vi "FGV.vi"(7 "State":enum16{"Set", "Get"}(ring)) -> (3 "Data Output":dbl)   [LabVIEW 2019]
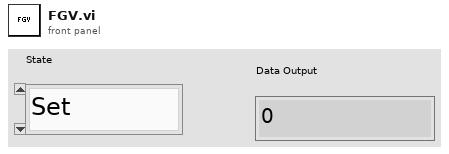
[diagram p1: front panel]
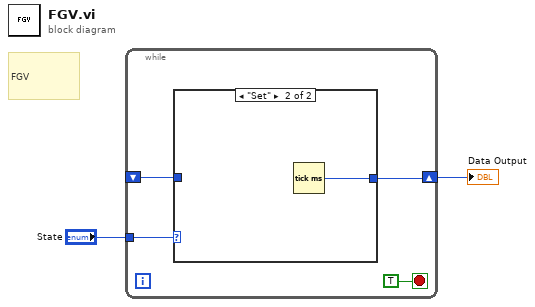
[diagram p0: block diagram]
diagram:
  # "FGV"
  n1 = while {
    shift-right: [w4] -> w1
    shift-left: _ -> [w3]
    tunnel: "State" -> [w5]
    stop <- TRUE stop-if-true
    n2 = case shown="\"Set\"" w5 {
      tunnel: [w7 w8] -> w4
      tunnel: w3 -> [w7 _]
      frame "Get" {
      }
      frame "Set" {
        n3 = Tick Count (ms)() -> (millisecond timer value=w8:u32)
      }
    }
  }
  "Data Output" <- w1
